vi "Save Settings.vi"(4 "error in (not an error)":errorcluster, 5 "channels":T2[](array[typedef]) {"input config" items=["no change", "differential", "ref. single-ended", "non-ref. single-ended", "4-wire"]; "coupling" items=["no change", "DC", "AC", "GND", "internal ref."]; "engineering units" items=["custom...", "V", "Pa", "g", "m/s^2", "m/s", "m", "in/s^2", "in/s", "in"]; "sensor sensitivity (mV/EU)" format="%.2f"; "range(+_)" format="%.2f"}, 6 "parameters":T1 {"Sample rate" format="%.2f"}, 7 "config file":path) -> (0 "error out":errorcluster, 3 "config file out":path)   [LabVIEW 2017]
uses:
  <vilib>/addons/Sound and Vibration/Order Analysis/Misc/OAT Channel Setting.ctl
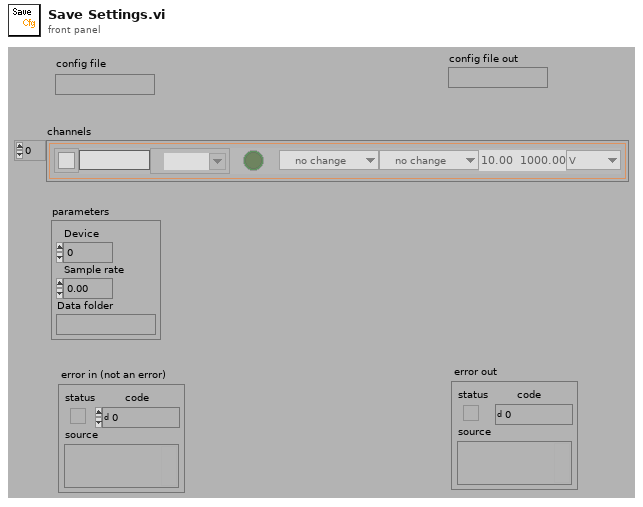
[diagram p1: front panel]
types:
  T1 = cluster{"Device":i16, "Sample rate":sgl, "Data folder":path}
  T2 = typedef "OAT Channel Setting.ctl" = cluster{"color":u32, "name":string, "channel":tag, "coupling":u16, "input config":u16, "range(+_)":sgl, "sensor sensitivity (mV/EU)":dbl, "engineering units":u16, "excitation":bool}
  T3 = enum16{"open", "open or create", "create or replace", "create"}
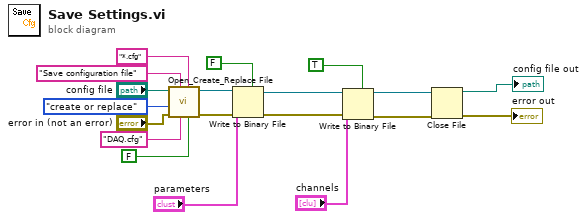
[diagram p0: block diagram]
diagram:
  n1 = call <vilib>:"Open_Create_Replace File.vi"("advisory dialog? (display:T)"=FALSE, "pattern"="*.cfg", "default name"="DAQ.cfg", "prompt"="Save configuration file", "error in (no error)"="error in (not an error)", "function (open:0)"=T3."create or replace", "file path"="config file") -> ("error out"=w18:errorcluster, "refnum"=w19:refnum<file>)  [unwired: 1 in, 2 out]
  n2 = Write to Binary File(file (use dialog)=w19, data="parameters", error in=w18, 5:FALSE ("prepend array or string size? (T)")) -> (refnum out=w17:refnum<file>, error out=w16:errorcluster)  [unwired: 2 in, 1 out]
  n3 = Write to Binary File(file (use dialog)=w17, data="channels", error in=w16, 5:TRUE ("header (F)")) -> (refnum out=w15:refnum<file>, error out=w14:errorcluster)  [unwired: 2 in, 1 out]
  n4 = Close File(refnum=w15, error in=w14) -> (path=→"config file out":path, error out=→"error out":errorcluster)
